vi "REACTOR_INICIA.vi"(8 "error in (no error)":errorcluster, 10 "ALICATS in":T1=[["A", "NO", "aM0000013", "Air", "100", "ln/mn", "0.1", "0.11"], ["B", "NO", "aM0000014", "Air", "100", "ln/mn", "0.2", "0.22"], ["C", "NO", "aM0000015", "Air", "100", "ln/mn", "0.3", "0.33"], ["D", "NO", "aM0000016", "Air", "500", "ln/mn", "0.4", "0.44"]] caption="Alicats", 11 "User event":T3) -> (0 "error out":errorcluster, 1 "ALICATS out":T1=[["A", "NO", "aM0000013", "Air", "100", "ln/mn", "0.1", "0.11"], ["B", "NO", "aM0000014", "Air", "100", "ln/mn", "0.2", "0.22"], ["C", "NO", "aM0000015", "Air", "100", "ln/mn", "0.3", "0.33"], ["D", "NO", "aM0000016", "Air", "500", "ln/mn", "0.4", "0.44"]] caption="Alicats", 3 "COMMS":T2={"Alicats"="ASRL6::INSTR", "Alic"=FALSE, "eValve"="ASRL6::INSTR", "eval"=FALSE, "Eurotherm"="ASRL6::INSTR", "euro"=FALSE, "Cell GAS"="ASRL6::INSTR", "cgas"=FALSE, "Cell H2S"="ASRL6::INSTR", "ch2s"=FALSE})   [LabVIEW 2017]
uses:
  DISPLAY/User Event Reference.ctl
  DISPLAY/User Event Data.ctl
  DISPLAY/Data Type.ctl
  REACTOR_COMUNICACIONES.ctl
  SERIAL ALICATS/__s_TablaAlicats.ctl
  DISPLAY/Display_Command Control.ctl
  EUROTHERM/Eurotherm_New_Module.ctl
  SERIAL RASP_PICO VALVE/kissia_rasPico Module.ctl
  SERIAL ALICATS/__Alicat SD_Hardware_Module.ctl
  REACTOR_GLOBALES.vi
panel:
  # "Aqui configuramos los parámetros de los ALICAT"
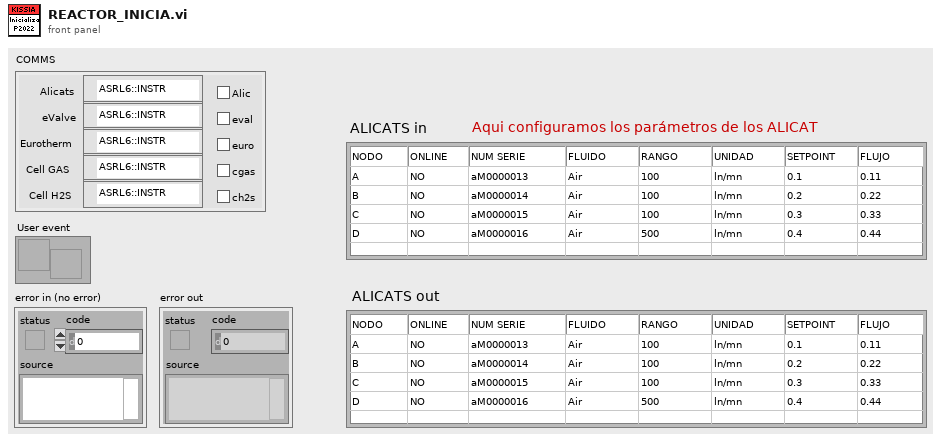
[diagram p1: front panel]
types:
  T1 = typedef "__s_TablaAlicats.ctl" = string[][]
  T2 = typedef "REACTOR_COMUNICACIONES.ctl" = cluster{"Alicats":refnum<visa-resource-name>, "Alic":bool, "eValve":refnum<visa-resource-name>, "eval":bool, "Eurotherm":refnum<visa-resource-name>, "euro":bool, "Cell GAS":refnum<visa-resource-name>, "cgas":bool, "Cell H2S":refnum<visa-resource-name>, "ch2s":bool}
  T3 = typedef "User Event Reference.ctl" = refnum<user-event>
  T4 = typedef "__Alicat SD_Hardware_Module.ctl" = enum16{"Initialize", "Send Setpoint", "Read Data", "Change Address", "Shutdown"}
  T5 = typedef "kissia_rasPico Module.ctl" = enum16{"Initialize", "Read Data", "Write Data", "Enable", "Disable", "Shutdown"}
  T6 = typedef "Eurotherm_New_Module.ctl" = enum16{"Initialize", "Write SP", "Read SP+PV", "Write Rate", "Set P", "Set I", "Set D", "Shutdown"}
  T7 = typedef "Data Type.ctl" = enum16{"Init FP", "En/Dis FP Ctls", "Update FP", "Upd Status", "Upd Seq"}
  T8 = typedef "Display_Command Control.ctl" = enum16{"Initialize", "Generate Event", "Shutdown"}
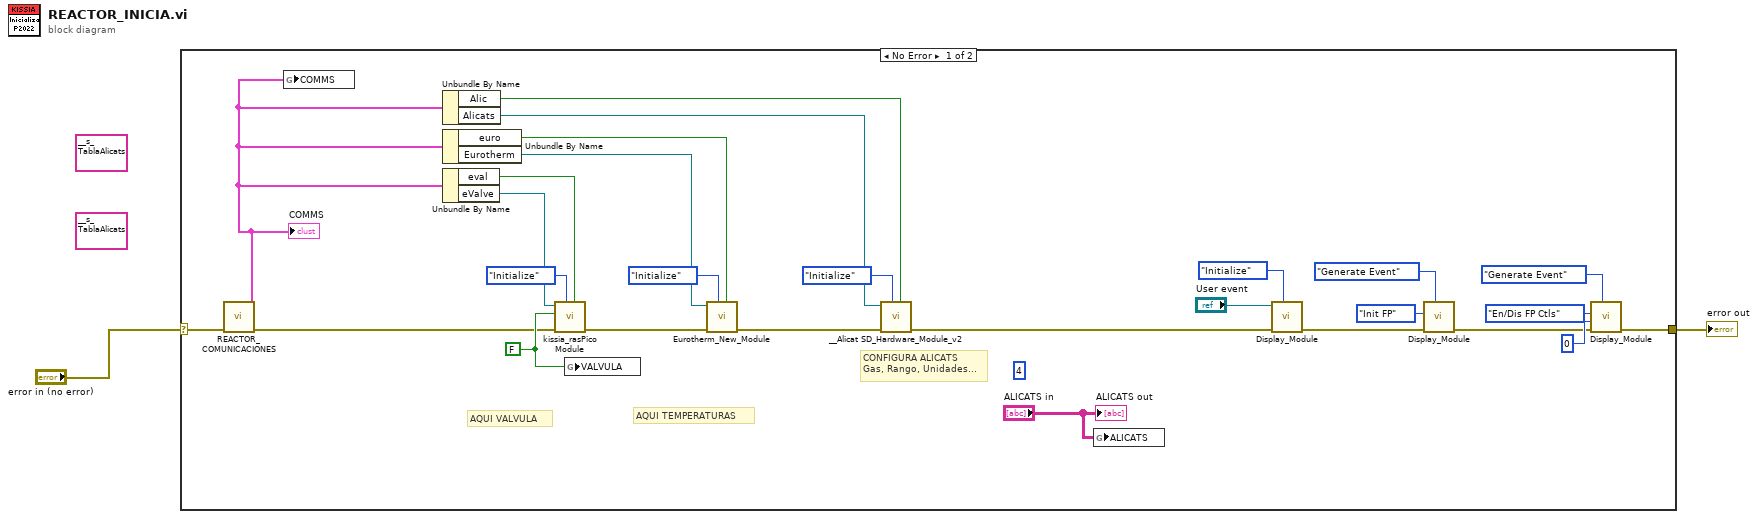
[diagram p0: block diagram]
diagram:
  (unwired) T1 [["3", "NO", "aM0000013", "Air", "1", "ln/mn", "0.1", "0.11"], ["4", "NO", "aM0000014", "Air", "1", "ln/mn", "0.2", "0.22"], ["5", "NO", "aM0000015", "Air", "1", "ln/mn", "0.3", "0.33"], ["6", "NO", "aM0000016", "Air", "1", "ln/mn", "0.4", "0.44"]] ("Dispositivos 2")
  (unwired) T1 [["3", "NO", "bM0000013", "Air", "1", "ln/mn", "0.1", "0.11"], ["4", "NO", "bM0000014", "Air", "1", "ln/mn", "0.2", "0.22"], ["5", "NO", "bM0000015", "Air", "1", "ln/mn", "0.3", "0.33"], ["6", "NO", "bM0000016", "Air", "1", "ln/mn", "0.4", "0.44"], ["7", "NO", "bM0000017", "Air", "1", "ln/mn", "0.5", "0.55"]] ("Dispositivos")
  n1 = case shown="No Error" "error in (no error)" {
    selector: "error in (no error)" -> [w25 w30]
    tunnel: [w11 w30] -> w1
    frame No Error {
      w17 = FALSE ("v5")
      (unwired) 4 ("Nodos")
      # "AQUI TEMPERATURAS"
      # "CONFIGURA ALICATS\nGas, Rango, Unidades..."
      # "AQUI VALVULA"
      n2 = call "REACTOR_COMUNICACIONES.vi"("error in (no error)"=w25) -> ("error out"=w10:errorcluster, "COMMS"=w14:T2)  [unwired: 8 in, 1 out]
      "COMMS" <- w14
      n3 = global write "REACTOR_GLOBALES.vi" "COMMS"(w14) -> ()
      n4 = Unbundle By Name(w14) -> ("Alic"=w5:bool, "Alicats"=w4:refnum<visa-resource-name>)
      n5 = Unbundle By Name(w14) -> ("euro"=w13:bool, "Eurotherm"=w12:refnum<visa-resource-name>)
      n6 = Unbundle By Name(w14) -> ("eval"=w19:bool, "eValve"=w18:refnum<visa-resource-name>)
      n7 = call "kissia_rasPico Module.vi"("Enable"=w19, "Command"=kissia_rasPico_Module."Initialize", "error in (no error)"=w10, "VALVE"=w17, "VISA resource name"=w18) -> ("error out"=w15:errorcluster)  [unwired: 3 in, 3 out]
      n8 = global write "REACTOR_GLOBALES.vi" "VALVULA"(w17) -> ()
      n9 = call "Eurotherm_New_Module.vi"("Eurotherm (T:Enable)"=w13, "Command"=Eurotherm_New_Module."Initialize", "error in (no error)"=w15, "VISA resource name"=w12) -> ("error out"=w8:errorcluster)  [unwired: 6 in, 1 out]
      n10 = call "__Alicat SD_Hardware_Module_v2.vi"("Used ?"=w5, "Command"=__Alicat_SD_Hardware_Module."Initialize", "error in (no error)"=w8, "VISA resource name"=w4) -> ("error out"=w7:errorcluster)  [unwired: 4 in, 3 out]
      n11 = global write "REACTOR_GLOBALES.vi" "ALICATS"("ALICATS in") -> ()
      n12 = call "Display_Module.vi"("Command"=Display_Command_Control."Initialize", "error in (no error)"=w7, "user event out"="User event") -> ("error out"=w27:errorcluster)  [unwired: 8 in]
      n13 = call "Display_Module.vi"("Command"=Display_Command_Control."Generate Event", "error in (no error)"=w27, "Data Type"=Data_Type."Init FP") -> ("error out"=w26:errorcluster)  [unwired: 8 in]
      n14 = call "Display_Module.vi"("Command"=Display_Command_Control."Generate Event", "error in (no error)"=w26, "Data"=0, "Data Type"=Data_Type."En/Dis FP Ctls") -> ("error out"=w11:errorcluster)  [unwired: 7 in]
      "ALICATS out" <- "ALICATS in"
    }
    frame Error {
    }
  }
  "error out" <- w1
